vi "Get Connected Entities.vi"(11 "terminal ref.":refnum<vi>) -> (1 "#terminals":i32, 3 "Connected Wire.Terminals[]":refnum<vi>[](array[refnum]))   [LabVIEW 2018]
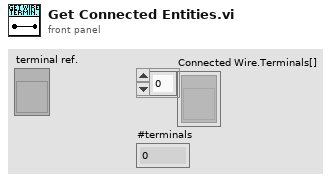
[diagram p1: front panel]
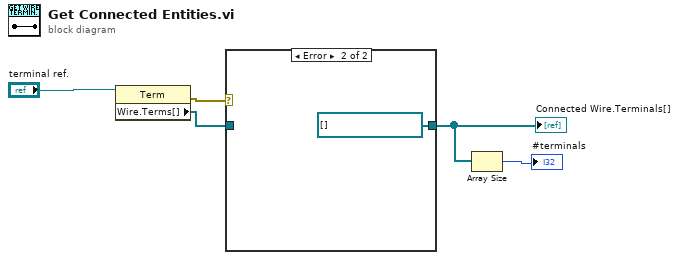
[diagram p0: block diagram]
diagram:
  n1 = property class="Term"(reference="terminal ref.") -> (error out=w4:errorcluster, "Wire.Terms[]"=w3:refnum<vi>[])  [unwired: 1 in, 1 out]
  n2 = case shown="Error" w4 {
    tunnel: [w6 refnum<vi>[] [] ("Wire.Terms[]")] -> w2
    tunnel: w3 -> [w6 _]
    frame No Error {
    }
    frame Error {
    }
  }
  "Connected Wire.Terminals[]" <- w2
  n3 = Array Size(array=w2) -> (size(s)=→"#terminals":i32)
